vi "normalizeAngle.vi"(11 "Input":dbl) -> (3 "Output":dbl)   [LabVIEW 2015]
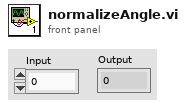
[diagram p1: front panel]
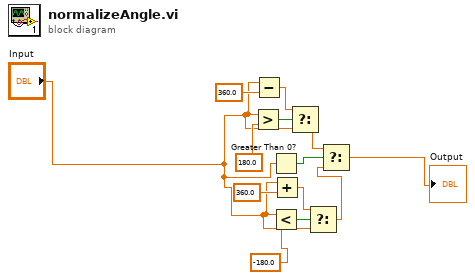
[diagram p0: block diagram]
diagram:
  n1 = Greater?(x="Input", y=180.0) -> (0:w12:bool)
  n2 = Subtract(x="Input", y=360.0) -> (x-y=w10:dbl)
  n3 = Greater Than 0?(x="Input") -> (x > 0?=w6:bool)
  n4 = Less?(x="Input", y=-180.0) -> (x < y?=w9:bool)
  n5 = Add(x="Input", y=360.0) -> (x+y=w7:dbl)
  n6 = Select(t=w10, s=w12, f="Input") -> (s? t:f=w5:dbl)
  n7 = Select(t=w7, s=w9, f="Input") -> (s? t:f=w1:dbl)
  n8 = Select(t=w5, s=w6, f=w1) -> (s? t:f=→"Output":dbl)
